vi "MD5 file.vi"(8 "error in (no error)":errorcluster, 10 "Path":path) -> (0 "error out":errorcluster, 2 "MD5 message-digest":string)   [LabVIEW 2016]
doc: "This VI computes the MD5 message-digest of a file, based on the algorithm described in RFC 1321 (http://www.ietf.org/rfc/rfc1321.txt). The MD5 message-digest is a 128-bit number, displayed in lower case hexadecimal."
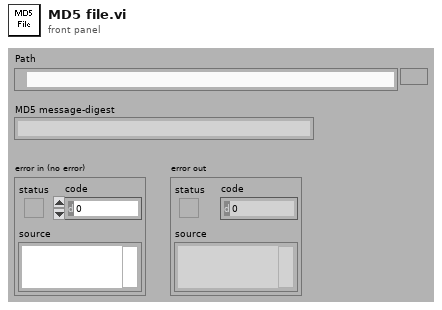
[diagram p1: front panel]
types:
  T1 = enum16{"open", "open or create", "create or replace", "create", "open (read only)"}
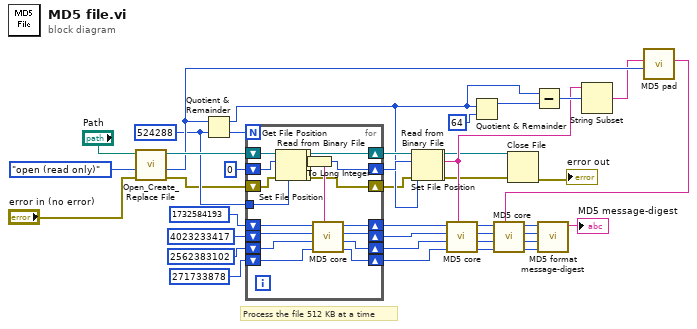
[diagram p0: block diagram]
diagram:
  w9 = 524288 ("y")
  # "Process the file 512 KB at a time"
  n1 = call <vilib>:"Open_Create_Replace File.vi"("error in (no error)"="error in (no error)", "function (open:0)"=T1."open (read only)", "file path"="Path") -> ("error out"=w4:errorcluster, "file size (bytes)"=w25:i32, "refnum"=w39:refnum<file>)  [unwired: 5 in, 1 out]
  n2 = Quotient & Remainder(x=w25, y=w9) -> (x-y*floor(x/y)=w10:i32, floor(x/y)=w38:i32)
  n3 = for {
    N: w38 -> [_]
    shift-right: [w56] -> w33
    shift-left: u32 1732584193 ("s1") -> [w61]
    shift-right: [w55] -> w32
    shift-left: u32 4023233417 ("s2") -> [w60]
    shift-right: [w54] -> w31
    shift-left: u32 2562383102 ("s3") -> [w59]
    shift-right: [w53] -> w30
    shift-left: u32 271733878 ("s4") -> [w58]
    shift-right: [w50] -> w27
    shift-left: 0 ("offset") -> [w51]
    tunnel: w9 -> [w49]
    shift-right: [w52] -> w28
    shift-left: w39 -> [w62]
    shift-right: [w47] -> w3
    shift-left: w4 -> [w48]
    n4 = Set File Position(offset (in bytes) (0)=w51, refnum=w62, error in=w48) -> (refnum out=w46:refnum<file>, error out=w45:errorcluster)  [unwired: 1 in]
    n5 = Read from Binary File(8:w45, 10:w49, 11:w46) -> (0:w43:errorcluster, 2:w57:string, 3:w44:refnum<file>)  [unwired: 3 in, 1 out]
    n6 = Get File Position(4:w43, 7:w44) -> (0:w47:errorcluster, 2:w42:i64, 3:w52:refnum<file>)
    n7 = To Long Integer(number=w42) -> (32bit integer=w50:i32)
    n8 = call "MD5 core.vi"("Input String"=w57, "s4"=w58, "s3"=w59, "s2"=w60, "s1"=w61) -> ("s4"=w53:u32, "s3"=w54:u32, "s2"=w55:u32, "s1"=w56:u32)  [unwired: 3 in]
  }
  n9 = Set File Position(offset (in bytes) (0)=w27, refnum=w28, error in=w3) -> (refnum out=w2:refnum<file>, error out=w1:errorcluster)  [unwired: 1 in]
  n10 = Read from Binary File(8:w1, 10:w10, 11:w2) -> (0:w7:errorcluster, 2:w11:string, 3:w8:refnum<file>)  [unwired: 3 in, 1 out]
  n11 = call "MD5 core.vi"("Input String"=w11, "s4"=w30, "s3"=w31, "s2"=w32, "s1"=w33) -> ("s4"=w18:u32, "s3"=w19:u32, "s2"=w20:u32, "s1"=w21:u32)  [unwired: 3 in]
  n12 = Quotient & Remainder(x=w10, y=64) -> (x-y*floor(x/y)=w24:i32)  [unwired: 1 out]
  n13 = Close File(refnum=w8, error in=w7) -> (error out=→"error out":errorcluster)  [unwired: 1 out]
  n14 = Subtract(x=w10, y=w24) -> (x-y=w23:i32)
  n15 = String Subset(string=w11, offset (0)=w23) -> (substring=w22:string)  [unwired: 1 in]
  n16 = call "MD5 pad.vi"("Message String Length (bytes)"=w25, "Last Part of Message String"=w22) -> ("Padding"=w17:string)  [unwired: 9 in]
  n17 = call "MD5 core.vi"("Input String"=w17, "s4"=w18, "s3"=w19, "s2"=w20, "s1"=w21) -> ("s4"=w13:u32, "s3"=w14:u32, "s2"=w15:u32, "s1"=w16:u32)  [unwired: 3 in]
  n18 = call "MD5 format message-digest.vi"("s4"=w13, "s3"=w14, "s2"=w15, "s1"=w16) -> ("MD5 message-digest"=→"MD5 message-digest":string)  [unwired: 7 in]
